vi "App - analyze RUS V6.vi"() -> ()   [LabVIEW 2021] (continued)
"mod time(min)"=58230516.86666667, "file format"=enum."binary", "power(V)"=2.1, "Magn Field(T) "=0.0}, {"temperature"=33.604, "temperature str"="33.60400", "file path"=path "D:/Data/Ultrasound/LSCO/LSCO22__130814c/5_Cooling_2nd_try/September_2014/091714/33.60400K_500_2500_2.10000V_0.00000T_Sep17-2014__16-38-11_001_091714.bin", "last mod"=timestamp(3493831091 s since 1904-01-01), "file name str"="D:\\Data\\Ultrasound\\LSCO\\LSCO22__130814c\\5_Cooling_2nd_try\\September_2014\\091714\\33.60400K_500_2500_2.10000V_0.00000T_Sep17-2014__16-38-11_001_091714.bin", "mod time(min)"=58230518.18333333, "file format"=enum."binary", "power(V)"=2.1, "Magn Field(T) "=0.0}, {"temperature"=33.517, "temperature str"="33.51700", "file path"=path "D:/Data/Ultrasound/LSCO/LSCO22__130814c/5_Cooling_2nd_try/September_2014/091714/33.51700K_500_2500_2.10000V_0.00000T_Sep17-2014__16-39-31_001_091714.bin", "last mod"=timestamp(3493831171 s since 1904-01-01), "file name str"="D:\\Data\\Ultrasound\\LSCO\\LSCO22__130814c\\5_Cooling_2nd_try\\September_2014\\091714\\33.51700K_500_2500_2.10000V_0.00000T_Sep17-2014__16-39-31_001_091714.bin", "mod time(min)"=58230519.516666666, "file format"=enum."binary", "power(V)"=2.1, "Magn Field(T) "=0.0}, {"temperature"=33.438, "temperature str"="33.43800", "file path"=path "D:/Data/Ultrasound/LSCO/LSCO22__130814c/5_Cooling_2nd_try/September_2014/091714/33.43800K_500_2500_2.10000V_0.00000T_Sep17-2014__16-40-50_001_091714.bin", "last mod"=timestamp(3493831250 s since 1904-01-01), "file name str"="D:\\Data\\Ultrasound\\LSCO\\LSCO22__130814c\\5_Cooling_2nd_try\\September_2014\\091714\\33.43800K_500_2500_2.10000V_0.00000T_Sep17-2014__16-40-50_001_091714.bin", "mod time(min)"=58230520.833333336, "file format"=enum."binary", "power(V)"=2.1, "Magn Field(T) "=0.0}, {"temperature"=33.342, "temperature str"="33.34200", "file path"=path "D:/Data/Ultrasound/LSCO/LSCO22__130814c/5_Cooling_2nd_try/September_2014/091714/33.34200K_500_2500_2.10000V_0.00000T_Sep17-2014__16-42-10_001_091714.bin", "last mod"=timestamp(3493831330 s since 1904-01-01), "file name str"="D:\\Data\\Ultrasound\\LSCO\\LSCO22__130814c\\5_Cooling_2nd_try\\September_2014\\091714\\33.34200K_500_2500_2.10000V_0.00000T_Sep17-2014__16-42-10_001_091714.bin", "mod time(min)"=58230522.166666664, "file format"=enum."binary", "power(V)"=2.1, "Magn Field(T) "=0.0}, {"temperature"=33.262, "temperature str"="33.26200", "file path"=path "D:/Data/Ultrasound/LSCO/LSCO22__130814c/5_Cooling_2nd_try/September_2014/091714/33.26200K_500_2500_2.10000V_0.00000T_Sep17-2014__16-43-29_001_091714.bin", "last mod"=timestamp(3493831409 s since 1904-01-01), "file name str"="D:\\Data\\Ultrasound\\LSCO\\LSCO22__130814c\\5_Cooling_2nd_try\\September_2014\\091714\\33.26200K_500_2500_2.10000V_0.00000T_Sep17-2014__16-43-29_001_091714.bin", "mod time(min)"=58230523.483333334, "file format"=enum."binary", "power(V)"=2.1, "Magn Field(T) "=0.0}, {"temperature"=33.17, "temperature str"="33.17000", "file path"=path "D:/Data/Ultrasound/LSCO/LSCO22__130814c/5_Cooling_2nd_try/September_2014/091714/33.17000K_500_2500_2.10000V_0.00000T_Sep17-2014__16-44-48_001_091714.bin", "last mod"=timestamp(3493831488 s since 1904-01-01), "file name str"="D:\\Data\\Ultrasound\\LSCO\\LSCO22__130814c\\5_Cooling_2nd_try\\September_2014\\091714\\33.17000K_500_2500_2.10000V_0.00000T_Sep17-2014__16-44-48_001_091714.bin", "mod time(min)"=58230524.8, "file format"=enum."binary", "power(V)"=2.1, "Magn Field(T) "=0.0}, {"temperature"=33.079, "temperature str"="33.07900", "file path"=path "D:/Data/Ultrasound/LSCO/LSCO22__130814c/5_Cooling_2nd_try/September_2014/091714/33.07900K_500_2500_2.10000V_0.00000T_Sep17-2014__16-46-08_001_091714.bin", "last mod"=timestamp(3493831568 s since 1904-01-01), "file name str"="D:\\Data\\Ultrasound\\LSCO\\LSCO22__130814c\\5_Cooling_2nd_try\\September_2014\\091714\\33.07900K_500_2500_2.10000V_0.00000T_Sep17-2014__16-46-08_001_091714.bin", "mod time(min)"=58230526.13333333, "file format"=enum."binary", "power(V)"=2.1, "Magn Field(T) "=0.0}, {"temperature"=32.992, "temperature str"="32.99200", "file path"=path "D:/Data/Ultrasound/LSCO/LSCO22__130814c/5_Cooling_2nd_try/September_2014/091714/32.99200K_500_2500_2.10000V_0.00000T_Sep17-2014__16-47-27_001_091714.bin", "last mod"=timestamp(3493831647 s since 1904-01-01), "file name str"="D:\\Data\\Ultrasound\\LSCO\\LSCO22__130814c\\5_Cooling_2nd_try\\September_2014\\091714\\32.99200K_500_2500_2.10000V_0.00000T_Sep17-2014__16-47-27_001_091714.bin", "mod time(min)"=58230527.45, "file format"=enum."binary", "power(V)"=2.1, "Magn Field(T) "=0.0}, {"temperature"=32.907, "temperature str"="32.90700", "file path"=path "D:/Data/Ultrasound/LSCO/LSCO22__130814c/5_Cooling_2nd_try/September_2014/091714/32.90700K_500_2500_2.10000V_0.00000T_Sep17-2014__16-48-46_001_091714.bin", "last mod"=timestamp(3493831726 s since 1904-01-01), "file name str"="D:\\Data\\Ultrasound\\LSCO\\LSCO22__130814c\\5_Cooling_2nd_try\\September_2014\\091714\\32.90700K_500_2500_2.10000V_0.00000T_Sep17-2014__16-48-46_001_091714.bin", "mod time(min)"=58230528.766666666, "file format"=enum."binary", "power(V)"=2.1, "Magn Field(T) "=0.0}, {"temperature"=32.817, "temperature str"="32.81700", "file path"=path "D:/Data/Ultrasound/LSCO/LSCO22__130814c/5_Cooling_2nd_try/September_2014/091714/32.81700K_500_2500_2.10000V_0.00000T_Sep17-2014__16-50-06_001_091714.bin", "last mod"=timestamp(3493831806 s since 1904-01-01), "file name str"="D:\\Data\\Ultrasound\\LSCO\\LSCO22__130814c\\5_Cooling_2nd_try\\September_2014\\091714\\32.81700K_500_2500_2.10000V_0.00000T_Sep17-2014__16-50-06_001_091714.bin", "mod time(min)"=58230530.1, "file format"=enum."binary", "power(V)"=2.1, "Magn Field(T) "=0.0}, {"temperature"=32.723, "temperature str"="32.72300", "file path"=path "D:/Data/Ultrasound/LSCO/LSCO22__130814c/5_Cooling_2nd_try/September_2014/091714/32.72300K_500_2500_2.10000V_0.00000T_Sep17-2014__16-51-25_001_091714.bin", "last mod"=timestamp(3493831885 s since 1904-01-01), "file name str"="D:\\Data\\Ultrasound\\LSCO\\LSCO22__130814c\\5_Cooling_2nd_try\\September_2014\\091714\\32.72300K_500_2500_2.10000V_0.00000T_Sep17-2014__16-51-25_001_091714.bin", "mod time(min)"=58230531.416666664, "file format"=enum."binary", "power(V)"=2.1, "Magn Field(T) "=0.0}, {"temperature"=32.637, "temperature str"="32.63700", "file path"=path "D:/Data/Ultrasound/LSCO/LSCO22__130814c/5_Cooling_2nd_try/September_2014/091714/32.63700K_500_2500_2.10000V_0.00000T_Sep17-2014__16-52-45_001_091714.bin", "last mod"=timestamp(3493831965 s since 1904-01-01), "file name str"="D:\\Data\\Ultrasound\\LSCO\\LSCO22__130814c\\5_Cooling_2nd_try\\September_2014\\091714\\32.63700K_500_2500_2.10000V_0.00000T_Sep17-2014__16-52-45_001_091714.bin", "mod time(min)"=58230532.75, "file format"=enum."binary", "power(V)"=2.1, "Magn Field(T) "=0.0}, {"temperature"=32.55, "temperature str"="32.55000", "file path"=path "D:/Data/Ultrasound/LSCO/LSCO22__130814c/5_Cooling_2nd_try/September_2014/091714/32.55000K_500_2500_2.10000V_0.00000T_Sep17-2014__16-54-04_001_091714.bin", "last mod"=timestamp(3493832044 s since 1904-01-01), "file name str"="D:\\Data\\Ultrasound\\LSCO\\LSCO22__130814c\\5_Cooling_2nd_try\\September_2014\\091714\\32.55000K_500_2500_2.10000V_0.00000T_Sep17-2014__16-54-04_001_091714.bin", "mod time(min)"=58230534.06666667, "file format"=enum."binary", "power(V)"=2.1, "Magn Field(T) "=0.0}, {"temperature"=32.462, "temperature str"="32.46200", "file path"=path "D:/Data/Ultrasound/LSCO/LSCO22__130814c/5_Cooling_2nd_try/September_2014/091714/32.46200K_500_2500_2.10000V_0.00000T_Sep17-2014__16-55-23_001_091714.bin", "last mod"=timestamp(3493832123 s since 1904-01-01), "file name str"="D:\\Data\\Ultrasound\\LSCO\\LSCO22__130814c\\5_Cooling_2nd_try\\September_2014\\091714\\32.46200K_500_2500_2.10000V_0.00000T_Sep17-2014__16-55-23_001_091714.bin", "mod time(min)"=58230535.38333333, "file format"=enum."binary", "power(V)"=2.1, "Magn Field(T) "=0.0}, {"temperature"=32.371, "temperature str"="32.37100", "file path"=path "D:/Data/Ultrasound/LSCO/LSCO22__130814c/5_Cooling_2nd_try/September_2014/091714/32.37100K_500_2500_2.10000V_0.00000T_Sep17-2014__16-56-43_001_091714.bin", "last mod"=timestamp(3493832203 s since 1904-01-01), "file name str"="D:\\Data\\Ultrasound\\LSCO\\LSCO22__130814c\\5_Cooling_2nd_try\\September_2014\\091714\\32.37100K_500_2500_2.10000V_0.00000T_Sep17-2014__16-56-43_001_091714.bin", "mod time(min)"=58230536.71666667, "file format"=enum."binary", "power(V)"=2.1, "Magn Field(T) "=0.0}, {"temperature"=32.282, "temperature str"="32.28200", "file path"=path "D:/Data/Ultrasound/LSCO/LSCO22__130814c/5_Cooling_2nd_try/September_2014/091714/32.28200K_500_2500_2.10000V_0.00000T_Sep17-2014__16-58-02_001_091714.bin", "last mod"=timestamp(3493832282 s since 1904-01-01), "file name str"="D:\\Data\\Ultrasound\\LSCO\\LSCO22__130814c\\5_Cooling_2nd_try\\September_2014\\091714\\32.28200K_500_2500_2.10000V_0.00000T_Sep17-2014__16-58-02_001_091714.bin", "mod time(min)"=58230538.03333333, "file format"=enum."binary", "power(V)"=2.1, "Magn Field(T) "=0.0}, {"temperature"=32.189, "temperature str"="32.18900", "file path"=path "D:/Data/Ultrasound/LSCO/LSCO22__130814c/5_Cooling_2nd_try/September_2014/091714/32.18900K_500_2500_2.10000V_0.00000T_Sep17-2014__16-59-22_001_091714.bin", "last mod"=timestamp(3493832362 s since 1904-01-01), "file name str"="D:\\Data\\Ultrasound\\LSCO\\LSCO22__130814c\\5_Cooling_2nd_try\\September_2014\\091714\\32.18900K_500_2500_2.10000V_0.00000T_Sep17-2014__16-59-22_001_091714.bin", "mod time(min)"=58230539.36666667, "file format"=enum."binary", "power(V)"=2.1, "Magn Field(T) "=0.0}, {"temperature"=32.102, "temperature str"="32.10200", "file path"=path "D:/Data/Ultrasound/LSCO/LSCO22__130814c/5_Cooling_2nd_try/September_2014/091714/32.10200K_500_2500_2.10000V_0.00000T_Sep17-2014__17-00-41_001_091714.bin", "last mod"=timestamp(3493832441 s since 1904-01-01), "file name str"="D:\\Data\\Ultrasound\\LSCO\\LSCO22__130814c\\5_Cooling_2nd_try\\September_2014\\091714\\32.10200K_500_2500_2.10000V_0.00000T_Sep17-2014__17-00-41_001_091714.bin", "mod time(min)"=58230540.68333333, "file format"=enum."binary", "power(V)"=2.1, "Magn Field(T) "=0.0}, {"temperature"=32.008, "temperature str"="32.00800", "file path"=path "D:/Data/Ultrasound/LSCO/LSCO22__130814c/5_Cooling_2nd_try/September_2014/091714/32.00800K_500_2500_2.10000V_0.00000T_Sep17-2014__17-02-00_001_091714.bin", "last mod"=timestamp(3493832520 s since 1904-01-01), "file name str"="D:\\Data\\Ultrasound\\LSCO\\LSCO22__130814c\\5_Cooling_2nd_try\\September_2014\\091714\\32.00800K_500_2500_2.10000V_0.00000T_Sep17-2014__17-02-00_001_091714.bin", "mod time(min)"=58230542.0, "file format"=enum."binary", "power(V)"=2.1, "Magn Field(T) "=0.0}, {"temperature"=31.925, "temperature str"="31.92500", "file path"=path "D:/Data/Ultrasound/LSCO/LSCO22__130814c/5_Cooling_2nd_try/September_2014/091714/31.92500K_500_2500_2.10000V_0.00000T_Sep17-2014__17-03-20_001_091714.bin", "last mod"=timestamp(3493832600 s since 1904-01-01), "file name str"="D:\\Data\\Ultrasound\\LSCO\\LSCO22__130814c\\5_Cooling_2nd_try\\September_2014\\091714\\31.92500K_500_2500_2.10000V_0.00000T_Sep17-2014__17-03-20_001_091714.bin", "mod time(min)"=58230543.333333336, "file format"=enum."binary", "power(V)"=2.1, "Magn Field(T) "=0.0}, {"temperature"=31.83, "temperature str"="31.83000", "file path"=path "D:/Data/Ultrasound/LSCO/LSCO22__130814c/5_Cooling_2nd_try/September_2014/091714/31.83000K_500_2500_2.10000V_0.00000T_Sep17-2014__17-04-39_001_091714.bin", "last mod"=timestamp(3493832679 s since 1904-01-01), "file name str"="D:\\Data\\Ultrasound\\LSCO\\LSCO22__130814c\\5_Cooling_2nd_try\\September_2014\\091714\\31.83000K_500_2500_2.10000V_0.00000T_Sep17-2014__17-04-39_001_091714.bin", "mod time(min)"=58230544.65, "file format"=enum."binary", "power(V)"=2.1, "Magn Field(T) "=0.0}, {"temperature"=31.738, "temperature str"="31.73800", "file path"=path "D:/Data/Ultrasound/LSCO/LSCO22__130814c/5_Cooling_2nd_try/September_2014/091714/31.73800K_500_2500_2.10000V_0.00000T_Sep17-2014__17-05-58_001_091714.bin", "last mod"=timestamp(3493832758 s since 1904-01-01), "file name str"="D:\\Data\\Ultrasound\\LSCO\\LSCO22__130814c\\5_Cooling_2nd_try\\September_2014\\091714\\31.73800K_500_2500_2.10000V_0.00000T_Sep17-2014__17-05-58_001_091714.bin", "mod time(min)"=58230545.96666667, "file format"=enum."binary", "power(V)"=2.1, "Magn Field(T) "=0.0}, {"temperature"=31.653, "temperature str"="31.65300", "file path"=path "D:/Data/Ultrasound/LSCO/LSCO22__130814c/5_Cooling_2nd_try/September_2014/091714/31.65300K_500_2500_2.10000V_0.00000T_Sep17-2014__17-07-18_001_091714.bin", "last mod"=timestamp(3493832838 s since 1904-01-01), "file name str"="D:\\Data\\Ultrasound\\LSCO\\LSCO22__130814c\\5_Cooling_2nd_try\\September_2014\\091714\\31.65300K_500_2500_2.10000V_0.00000T_Sep17-2014__17-07-18_001_091714.bin", "mod time(min)"=58230547.3, "file format"=enum."binary", "power(V)"=2.1, "Magn Field(T) "=0.0}, {"temperature"=31.556, "temperature str"="31.55600", "file path"=path "D:/Data/Ultrasound/LSCO/LSCO22__130814c/5_Cooling_2nd_try/September_2014/091714/31.55600K_500_2500_2.10000V_0.00000T_Sep17-2014__17-08-37_001_091714.bin", "last mod"=timestamp(3493832917 s since 1904-01-01), "file name str"="D:\\Data\\Ultrasound\\LSCO\\LSCO22__130814c\\5_Cooling_2nd_try\\September_2014\\091714\\31.55600K_500_2500_2.10000V_0.00000T_Sep17-2014__17-08-37_001_091714.bin", "mod time(min)"=58230548.61666667, "file format"=enum."binary", "power(V)"=2.1, "Magn Field(T) "=0.0}, {"temperature"=31.463, "temperature str"="31.46300", "file path"=path "D:/Data/Ultrasound/LSCO/LSCO22__130814c/5_Cooling_2nd_try/September_2014/091714/31.46300K_500_2500_2.10000V_0.00000T_Sep17-2014__17-09-57_001_091714.bin", "last mod"=timestamp(3493832997 s since 1904-01-01), "file name str"="D:\\Data\\Ultrasound\\LSCO\\LSCO22__130814c\\5_Cooling_2nd_try\\September_2014\\091714\\31.46300K_500_2500_2.10000V_0.00000T_Sep17-2014__17-09-57_001_091714.bin", "mod time(min)"=58230549.95, "file format"=enum."binary", "power(V)"=2.1, "Magn Field(T) "=0.0}, {"temperature"=31.383, "temperature str"="31.38300", "file path"=path "D:/Data/Ultrasound/LSCO/LSCO22__130814c/5_Cooling_2nd_try/September_2014/091714/31.38300K_500_2500_2.10000V_0.00000T_Sep17-2014__17-11-16_001_091714.bin", "last mod"=timestamp(3493833076 s since 1904-01-01), "file name str"="D:\\Data\\Ultrasound\\LSCO\\LSCO22__130814c\\5_Cooling_2nd_try\\September_2014\\091714\\31.38300K_500_2500_2.10000V_0.00000T_Sep17-2014__17-11-16_001_091714.bin", "mod time(min)"=58230551.266666666, "file format"=enum."binary", "power(V)"=2.1, "Magn Field(T) "=0.0}, {"temperature"=31.282, "temperature str"="31.28200", "file path"=path "D:/Data/Ultrasound/LSCO/LSCO22__130814c/5_Cooling_2nd_try/September_2014/091714/31.28200K_500_2500_2.10000V_0.00000T_Sep17-2014__17-12-35_001_091714.bin", "last mod"=timestamp(3493833155 s since 1904-01-01), "file name str"="D:\\Data\\Ultrasound\\LSCO\\LSCO22__130814c\\5_Cooling_2nd_try\\September_2014\\091714\\31.28200K_500_2500_2.10000V_0.00000T_Sep17-2014__17-12-35_001_091714.bin", "mod time(min)"=58230552.583333336, "file format"=enum."binary", "power(V)"=2.1, "Magn Field(T) "=0.0}, {"temperature"=31.196, "temperature str"="31.19600", "file path"=path "D:/Data/Ultrasound/LSCO/LSCO22__130814c/5_Cooling_2nd_try/September_2014/091714/31.19600K_500_2500_2.10000V_0.00000T_Sep17-2014__17-13-55_001_091714.bin", "last mod"=timestamp(3493833235 s since 1904-01-01), "file name str"="D:\\Data\\Ultrasound\\LSCO\\LSCO22__130814c\\5_Cooling_2nd_try\\September_2014\\091714\\31.19600K_500_2500_2.10000V_0.00000T_Sep17-2014__17-13-55_001_091714.bin", "mod time(min)"=58230553.916666664, "file format"=enum."binary", "power(V)"=2.1, "Magn Field(T) "=0.0}, {"temperature"=31.111, "temperature str"="31.11100", "file path"=path "D:/Data/Ultrasound/LSCO/LSCO22__130814c/5_Cooling_2nd_try/September_2014/091714/31.11100K_500_2500_2.10000V_0.00000T_Sep17-2014__17-15-14_001_091714.bin", "last mod"=timestamp(3493833314 s since 1904-01-01), "file name str"="D:\\Data\\Ultrasound\\LSCO\\LSCO22__130814c\\5_Cooling_2nd_try\\September_2014\\091714\\31.11100K_500_2500_2.10000V_0.00000T_Sep17-2014__17-15-14_001_091714.bin", "mod time(min)"=58230555.233333334, "file format"=enum."binary", "power(V)"=2.1, "Magn Field(T) "=0.0}, {"temperature"=31.006, "temperature str"="31.00600", "file path"=path "D:/Data/Ultrasound/LSCO/LSCO22__130814c/5_Cooling_2nd_try/September_2014/091714/31.00600K_500_2500_2.10000V_0.00000T_Sep17-2014__17-16-33_001_091714.bin", "last mod"=timestamp(3493833393 s since 1904-01-01), "file name str"="D:\\Data\\Ultrasound\\LSCO\\LSCO22__130814c\\5_Cooling_2nd_try\\September_2014\\091714\\31.00600K_500_2500_2.10000V_0.00000T_Sep17-2014__17-16-33_001_091714.bin", "mod time(min)"=58230556.55, "file format"=enum."binary", "power(V)"=2.1, "Magn Field(T) "=0.0}, {"temperature"=30.926, "temperature str"="30.92600", "file path"=path "D:/Data/Ultrasound/LSCO/LSCO22__130814c/5_Cooling_2nd_try/September_2014/091714/30.92600K_500_2500_2.10000V_0.00000T_Sep17-2014__17-17-53_001_091714.bin", "last mod"=timestamp(3493833473 s since 1904-01-01), "file name str"="D:\\Data\\Ultrasound\\LSCO\\LSCO22__130814c\\5_Cooling_2nd_try\\September_2014\\091714\\30.92600K_500_2500_2.10000V_0.00000T_Sep17-2014__17-17-53_001_091714.bin", "mod time(min)"=58230557.88333333, "file format"=enum."binary", "power(V)"=2.1, "Magn Field(T) "=0.0}, {"temperature"=30.834, "temperature str"="30.83400", "file path"=path "D:/Data/Ultrasound/LSCO/LSCO22__130814c/5_Cooling_2nd_try/September_2014/091714/30.83400K_500_2500_2.10000V_0.00000T_Sep17-2014__17-19-12_001_091714.bin", "last mod"=timestamp(3493833552 s since 1904-01-01), "file name str"="D:\\Data\\Ultrasound\\LSCO\\LSCO22__130814c\\5_Cooling_2nd_try\\September_2014\\091714\\30.83400K_500_2500_2.10000V_0.00000T_Sep17-2014__17-19-12_001_091714.bin", "mod time(min)"=58230559.2, "file format"=enum."binary", "power(V)"=2.1, "Magn Field(T) "=0.0}, {"temperature"=30.738, "temperature str"="30.73800", "file path"=path "D:/Data/Ultrasound/LSCO/LSCO22__130814c/5_Cooling_2nd_try/September_2014/091714/30.73800K_500_2500_2.10000V_0.00000T_Sep17-2014__17-20-32_001_091714.bin", "last mod"=timestamp(3493833632 s since 1904-01-01), "file name str"="D:\\Data\\Ultrasound\\LSCO\\LSCO22__130814c\\5_Cooling_2nd_try\\September_2014\\091714\\30.73800K_500_2500_2.10000V_0.00000T_Sep17-2014__17-20-32_001_091714.bin", "mod time(min)"=58230560.53333333, "file format"=enum."binary", "power(V)"=2.1, "Magn Field(T) "=0.0}, {"temperature"=30.648, "temperature str"="30.64800", "file path"=path "D:/Data/Ultrasound/LSCO/LSCO22__130814c/5_Cooling_2nd_try/September_2014/091714/30.64800K_500_2500_2.10000V_0.00000T_Sep17-2014__17-21-51_001_091714.bin", "last mod"=timestamp(3493833711 s since 1904-01-01), "file name str"="D:\\Data\\Ultrasound\\LSCO\\LSCO22__130814c\\5_Cooling_2nd_try\\September_2014\\091714\\30.64800K_500_2500_2.10000V_0.00000T_Sep17-2014__17-21-51_001_091714.bin", "mod time(min)"=58230561.85, "file format"=enum."binary", "power(V)"=2.1, "Magn Field(T) "=0.0}, {"temperature"=30.563, "temperature str"="30.56300", "file path"=path "D:/Data/Ultrasound/LSCO/LSCO22__130814c/5_Cooling_2nd_try/September_2014/091714/30.56300K_500_2500_2.10000V_0.00000T_Sep17-2014__17-23-10_001_091714.bin", "last mod"=timestamp(3493833790 s since 1904-01-01), "file name str"="D:\\Data\\Ultrasound\\LSCO\\LSCO22__130814c\\5_Cooling_2nd_try\\September_2014\\091714\\30.56300K_500_2500_2.10000V_0.00000T_Sep17-2014__17-23-10_001_091714.bin", "mod time(min)"=58230563.166666664, "file format"=enum."binary", "power(V)"=2.1, "Magn Field(T) "=0.0}, {"temperature"=30.467, "temperature str"="30.46700", "file path"=path "D:/Data/Ultrasound/LSCO/LSCO22__130814c/5_Cooling_2nd_try/September_2014/091714/30.46700K_500_2500_2.10000V_0.00000T_Sep17-2014__17-24-30_001_091714.bin", "last mod"=timestamp(3493833870 s since 1904-01-01), "file name str"="D:\\Data\\Ultrasound\\LSCO\\LSCO22__130814c\\5_Cooling_2nd_try\\September_2014\\091714\\30.46700K_500_2500_2.10000V_0.00000T_Sep17-2014__17-24-30_001_091714.bin", "mod time(min)"=58230564.5, "file format"=enum."binary", "power(V)"=2.1, "Magn Field(T) "=0.0}, {"temperature"=30.376, "temperature str"="30.37600", "file path"=path "D:/Data/Ultrasound/LSCO/LSCO22__130814c/5_Cooling_2nd_try/September_2014/091714/30.37600K_500_2500_2.10000V_0.00000T_Sep17-2014__17-25-49_001_091714.bin", "last mod"=timestamp(3493833949 s since 1904-01-01), "file name str"="D:\\Data\\Ultrasound\\LSCO\\LSCO22__130814c\\5_Cooling_2nd_try\\September_2014\\091714\\30.37600K_500_2500_2.10000V_0.00000T_Sep17-2014__17-25-49_001_091714.bin", "mod time(min)"=58230565.81666667, "file format"=enum."binary", "power(V)"=2.1, "Magn Field(T) "=0.0}, {"temperature"=30.285, "temperature str"="30.28500", "file path"=path "D:/Data/Ultrasound/LSCO/LSCO22__130814c/5_Cooling_2nd_try/September_2014/091714/30.28500K_500_2500_2.10000V_0.00000T_Sep17-2014__17-27-09_001_091714.bin", "last mod"=timestamp(3493834029 s since 1904-01-01), "file name str"="D:\\Data\\Ultrasound\\LSCO\\LSCO22__130814c\\5_Cooling_2nd_try\\September_2014\\091714\\30.28500K_500_2500_2.10000V_0.00000T_Sep17-2014__17-27-09_001_091714.bin", "mod time(min)"=58230567.15, "file format"=enum."binary", "power(V)"=2.1, "Magn Field(T) "=0.0}, {"temperature"=30.196, "temperature str"="30.19600", "file path"=path "D:/Data/Ultrasound/LSCO/LSCO22__130814c/5_Cooling_2nd_try/September_2014/091714/30.19600K_500_2500_2.10000V_0.00000T_Sep17-2014__17-28-28_001_091714.bin", "last mod"=timestamp(3493834108 s since 1904-01-01), "file name str"="D:\\Data\\Ultrasound\\LSCO\\LSCO22__130814c\\5_Cooling_2nd_try\\September_2014\\091714\\30.19600K_500_2500_2.10000V_0.00000T_Sep17-2014__17-28-28_001_091714.bin", "mod time(min)"=58230568.46666667, "file format"=enum."binary", "power(V)"=2.1, "Magn Field(T) "=0.0}, {"temperature"=30.104, "temperature str"="30.10400", "file path"=path "D:/Data/Ultrasound/LSCO/LSCO22__130814c/5_Cooling_2nd_try/September_2014/091714/30.10400K_500_2500_2.10000V_0.00000T_Sep17-2014__17-29-47_001_091714.bin", "last mod"=timestamp(3493834187 s since 1904-01-01), "file name str"="D:\\Data\\Ultrasound\\LSCO\\LSCO22__130814c\\5_Cooling_2nd_try\\September_2014\\091714\\30.10400K_500_2500_2.10000V_0.00000T_Sep17-2014__17-29-47_001_091714.bin", "mod time(min)"=58230569.78333333, "file format"=enum."binary", "power(V)"=2.1, "Magn Field(T) "=0.0}, {"temperature"=30.009, "temperature str"="30.00900", "file path"=path "D:/Data/Ultrasound/LSCO/LSCO22__130814c/5_Cooling_2nd_try/September_2014/091714/30.00900K_500_2500_2.10000V_0.00000T_Sep17-2014__17-31-07_001_091714.bin", "last mod"=timestamp(3493834267 s since 1904-01-01), "file name str"="D:\\Data\\Ultrasound\\LSCO\\LSCO22__130814c\\5_Cooling_2nd_try\\September_2014\\091714\\30.00900K_500_2500_2.10000V_0.00000T_Sep17-2014__17-31-07_001_091714.bin", "mod time(min)"=58230571.11666667, "file format"=enum."binary", "power(V)"=2.1, "Magn Field(T) "=0.0}, {"temperature"=29.914, "temperature str"="29.91400", "file path"=path "D:/Data/Ultrasound/LSCO/LSCO22__130814c/5_Cooling_2nd_try/September_2014/091714/29.91400K_500_2500_2.10000V_0.00000T_Sep17-2014__17-32-26_001_091714.bin", "last mod"=timestamp(3493834346 s since 1904-01-01), "file name str"="D:\\Data\\Ultrasound\\LSCO\\LSCO22__130814c\\5_Cooling_2nd_try\\September_2014\\091714\\29.91400K_500_2500_2.10000V_0.00000T_Sep17-2014__17-32-26_001_091714.bin", "mod time(min)"=58230572.43333333, "file format"=enum."binary", "power(V)"=2.1, "Magn Field(T) "=0.0}, {"temperature"=29.832, "temperature str"="29.83200", "file path"=path "D:/Data/Ultrasound/LSCO/LSCO22__130814c/5_Cooling_2nd_try/September_2014/091714/29.83200K_500_2500_2.10000V_0.00000T_Sep17-2014__17-33-45_001_091714.bin", "last mod"=timestamp(3493834425 s since 1904-01-01), "file name str"="D:\\Data\\Ultrasound\\LSCO\\LSCO22__130814c\\5_Cooling_2nd_try\\September_2014\\091714\\29.83200K_500_2500_2.10000V_0.00000T_Sep17-2014__17-33-45_001_091714.bin", "mod time(min)"=58230573.75, "file format"=enum."binary", "power(V)"=2.1, "Magn Field(T) "=0.0}, {"temperature"=29.737, "temperature str"="29.73700", "file path"=path "D:/Data/Ultrasound/LSCO/LSCO22__130814c/5_Cooling_2nd_try/September_2014/091714/29.73700K_500_2500_2.10000V_0.00000T_Sep17-2014__17-35-05_001_091714.bin", "last mod"=timestamp(3493834505 s since 1904-01-01), "file name str"="D:\\Data\\Ultrasound\\LSCO\\LSCO22__130814c\\5_Cooling_2nd_try\\September_2014\\091714\\29.73700K_500_2500_2.10000V_0.00000T_Sep17-2014__17-35-05_001_091714.bin", "mod time(min)"=58230575.083333336, "file format"=enum."binary", "power(V)"=2.1, "Magn Field(T) "=0.0}, {"temperature"=29.637, "temperature str"="29.63700", "file path"=path "D:/Data/Ultrasound/LSCO/LSCO22__130814c/5_Cooling_2nd_try/September_2014/091714/29.63700K_500_2500_2.10000V_0.00000T_Sep17-2014__17-36-24_001_091714.bin", "last mod"=timestamp(3493834584 s since 1904-01-01), "file name str"="D:\\Data\\Ultrasound\\LSCO\\LSCO22__130814c\\5_Cooling_2nd_try\\September_2014\\091714\\29.63700K_500_2500_2.10000V_0.00000T_Sep17-2014__17-36-24_001_091714.bin", "mod time(min)"=58230576.4, "file format"=enum."binary", "power(V)"=2.1, "Magn Field(T) "=0.0}, {"temperature"=29.553, "temperature str"="29.55300", "file path"=path "D:/Data/Ultrasound/LSCO/LSCO22__130814c/5_Cooling_2nd_try/September_2014/091714/29.55300K_500_2500_2.10000V_0.00000T_Sep17-2014__17-37-44_001_091714.bin", "last mod"=timestamp(3493834664 s since 1904-01-01), "file name str"="D:\\Data\\Ultrasound\\LSCO\\LSCO22__130814c\\5_Cooling_2nd_try\\September_2014\\091714\\29.55300K_500_2500_2.10000V_0.00000T_Sep17-2014__17-37-44_001_091714.bin", "mod time(min)"=58230577.733333334, "file format"=enum."binary", "power(V)"=2.1, "Magn Field(T) "=0.0}, {"temperature"=29.453, "temperature str"="29.45300", "file path"=path "D:/Data/Ultrasound/LSCO/LSCO22__130814c/5_Cooling_2nd_try/September_2014/091714/29.45300K_500_2500_2.10000V_0.00000T_Sep17-2014__17-39-03_001_091714.bin", "last mod"=timestamp(3493834743 s since 1904-01-01), "file name str"="D:\\Data\\Ultrasound\\LSCO\\LSCO22__130814c\\5_Cooling_2nd_try\\September_2014\\091714\\29.45300K_500_2500_2.10000V_0.00000T_Sep17-2014__17-39-03_001_091714.bin", "mod time(min)"=58230579.05, "file format"=enum."binary", "power(V)"=2.1, "Magn Field(T) "=0.0}, {"temperature"=29.362, "temperature str"="29.36200", "file path"=path "D:/Data/Ultrasound/LSCO/LSCO22__130814c/5_Cooling_2nd_try/September_2014/091714/29.36200K_500_2500_2.10000V_0.00000T_Sep17-2014__17-40-22_001_091714.bin", "last mod"=timestamp(3493834822 s since 1904-01-01), "file name str"="D:\\Data\\Ultrasound\\LSCO\\LSCO22__130814c\\5_Cooling_2nd_try\\September_2014\\091714\\29.36200K_500_2500_2.10000V_0.00000T_Sep17-2014__17-40-22_001_091714.bin", "mod time(min)"=58230580.36666667, "file format"=enum."binary", "power(V)"=2.1, "Magn Field(T) "=0.0}, {"temperature"=29.272, "temperature str"="29.27200", "file path"=path "D:/Data/Ultrasound/LSCO/LSCO22__130814c/5_Cooling_2nd_try/September_2014/091714/29.27200K_500_2500_2.10000V_0.00000T_Sep17-2014__17-41-42_001_091714.bin", "last mod"=timestamp(3493834902 s since 1904-01-01), "file name str"="D:\\Data\\Ultrasound\\LSCO\\LSCO22__130814c\\5_Cooling_2nd_try\\September_2014\\091714\\29.27200K_500_2500_2.10000V_0.00000T_Sep17-2014__17-41-42_001_091714.bin", "mod time(min)"=58230581.7, "file format"=enum."binary", "power(V)"=2.1, "Magn Field(T) "=0.0}, {"temperature"=29.18, "temperature str"="29.18000", "file path"=path "D:/Data/Ultrasound/LSCO/LSCO22__130814c/5_Cooling_2nd_try/September_2014/091714/29.18000K_500_2500_2.10000V_0.00000T_Sep17-2014__17-43-01_001_091714.bin", "last mod"=timestamp(3493834981 s since 1904-01-01), "file name str"="D:\\Data\\Ultrasound\\LSCO\\LSCO22__130814c\\5_Cooling_2nd_try\\September_2014\\091714\\29.18000K_500_2500_2.10000V_0.00000T_Sep17-2014__17-43-01_001_091714.bin", "mod time(min)"=58230583.016666666, "file format"=enum."binary", "power(V)"=2.1, "Magn Field(T) "=0.0}, {"temperature"=29.085, "temperature str"="29.08500", "file path"=path "D:/Data/Ultrasound/LSCO/LSCO22__130814c/5_Cooling_2nd_try/September_2014/091714/29.08500K_500_2500_2.10000V_0.00000T_Sep17-2014__17-44-21_001_091714.bin", "last mod"=timestamp(3493835061 s since 1904-01-01), "file name str"="D:\\Data\\Ultrasound\\LSCO\\LSCO22__130814c\\5_Cooling_2nd_try\\September_2014\\091714\\29.08500K_500_2500_2.10000V_0.00000T_Sep17-2014__17-44-21_001_091714.bin", "mod time(min)"=58230584.35, "file format"=enum."binary", "power(V)"=2.1, "Magn Field(T) "=0.0}, {"temperature"=28.992, "temperature str"="28.99200", "file path"=path "D:/Data/Ultrasound/LSCO/LSCO22__130814c/5_Cooling_2nd_try/September_2014/091714/28.99200K_500_2500_2.10000V_0.00000T_Sep17-2014__17-45-40_001_091714.bin", "last mod"=timestamp(3493835140 s since 1904-01-01), "file name str"="D:\\Data\\Ultrasound\\LSCO\\LSCO22__130814c\\5_Cooling_2nd_try\\September_2014\\091714\\28.99200K_500_2500_2.10000V_0.00000T_Sep17-2014__17-45-40_001_091714.bin", "mod time(min)"=58230585.666666664, "file format"=enum."binary", "power(V)"=2.1, "Magn Field(T) "=0.0}, {"temperature"=28.892, "temperature str"="28.89200", "file path"=path "D:/Data/Ultrasound/LSCO/LSCO22__130814c/5_Cooling_2nd_try/September_2014/091714/28.89200K_500_2500_2.10000V_0.00000T_Sep17-2014__17-46-59_001_091714.bin", "last mod"=timestamp(3493835219 s since 1904-01-01), "file name str"="D:\\Data\\Ultrasound\\LSCO\\LSCO22__130814c\\5_Cooling_2nd_try\\September_2014\\091714\\28.89200K_500_2500_2.10000V_0.00000T_Sep17-2014__17-46-59_001_091714.bin", "mod time(min)"=58230586.983333334, "file format"=enum."binary", "power(V)"=2.1, "Magn Field(T) "=0.0}, {"temperature"=28.803, "temperature str"="28.80300", "file path"=path "D:/Data/Ultrasound/LSCO/LSCO22__130814c/5_Cooling_2nd_try/September_2014/091714/28.80300K_500_2500_2.10000V_0.00000T_Sep17-2014__17-48-19_001_091714.bin", "last mod"=timestamp(3493835299 s since 1904-01-01), "file name str"="D:\\Data\\Ultrasound\\LSCO\\LSCO22__130814c\\5_Cooling_2nd_try\\September_2014\\091714\\28.80300K_500_2500_2.10000V_0.00000T_Sep17-2014__17-48-19_001_091714.bin", "mod time(min)"=58230588.31666667, "file format"=enum."binary", "power(V)"=2.1, "Magn Field(T) "=0.0}, {"temperature"=28.71, "temperature str"="28.71000", "file path"=path "D:/Data/Ultrasound/LSCO/LSCO22__130814c/5_Cooling_2nd_try/September_2014/091714/28.71000K_500_2500_2.10000V_0.00000T_Sep17-2014__17-49-38_001_091714.bin", "last mod"=timestamp(3493835378 s since 1904-01-01), "file name str"="D:\\Data\\Ultrasound\\LSCO\\LSCO22__130814c\\5_Cooling_2nd_try\\September_2014\\091714\\28.71000K_500_2500_2.10000V_0.00000T_Sep17-2014__17-49-38_001_091714.bin", "mod time(min)"=58230589.63333333, "file format"=enum."binary", "power(V)"=2.1, "Magn Field(T) "=0.0}, {"temperature"=28.614, "temperature str"="28.61400", "file path"=path "D:/Data/Ultrasound/LSCO/LSCO22__130814c/5_Cooling_2nd_try/September_2014/091714/28.61400K_500_2500_2.10000V_0.00000T_Sep17-2014__17-50-57_001_091714.bin", "last mod"=timestamp(3493835457 s since 1904-01-01), "file name str"="D:\\Data\\Ultrasound\\LSCO\\LSCO22__130814c\\5_Cooling_2nd_try\\September_2014\\091714\\28.61400K_500_2500_2.10000V_0.00000T_Sep17-2014__17-50-57_001_091714.bin", "mod time(min)"=58230590.95, "file format"=enum."binary", "power(V)"=2.1, "Magn Field(T) "=0.0}, {"temperature"=28.52, "temperature str"="28.52000", "file path"=path "D:/Data/Ultrasound/LSCO/LSCO22__130814c/5_Cooling_2nd_try/September_2014/091714/28.52000K_500_2500_2.10000V_0.00000T_Sep17-2014__17-52-17_001_091714.bin", "last mod"=timestamp(3493835537 s since 1904-01-01), "file name str"="D:\\Data\\Ultrasound\\LSCO\\LSCO22__130814c\\5_Cooling_2nd_try\\September_2014\\091714\\28.52000K_500_2500_2.10000V_0.00000T_Sep17-2014__17-52-17_001_091714.bin", "mod time(min)"=58230592.28333333, "file format"=enum."binary", "power(V)"=2.1, "Magn Field(T) "=0.0}, {"temperature"=28.426, "temperature str"="28.42600", "file path"=path "D:/Data/Ultrasound/LSCO/LSCO22__130814c/5_Cooling_2nd_try/September_2014/091714/28.42600K_500_2500_2.10000V_0.00000T_Sep17-2014__17-53-36_001_091714.bin", "last mod"=timestamp(3493835616 s since 1904-01-01), "file name str"="D:\\Data\\Ultrasound\\LSCO\\LSCO22__130814c\\5_Cooling_2nd_try\\September_2014\\091714\\28.42600K_500_2500_2.10000V_0.00000T_Sep17-2014__17-53-36_001_091714.bin", "mod time(min)"=58230593.6, "file format"=enum."binary", "power(V)"=2.1, "Magn Field(T) "=0.0}, {"temperature"=28.336, "temperature str"="28.33600", "file path"=path "D:/Data/Ultrasound/LSCO/LSCO22__130814c/5_Cooling_2nd_try/September_2014/091714/28.33600K_500_2500_2.10000V_0.00000T_Sep17-2014__17-54-56_001_091714.bin", "last mod"=timestamp(3493835696 s since 1904-01-01), "file name str"="D:\\Data\\Ultrasound\\LSCO\\LSCO22__130814c\\5_Cooling_2nd_try\\September_2014\\091714\\28.33600K_500_2500_2.10000V_0.00000T_Sep17-2014__17-54-56_001_091714.bin", "mod time(min)"=58230594.93333333, "file format"=enum."binary", "power(V)"=2.1, "Magn Field(T) "=0.0}, {"temperature"=28.239, "temperature str"="28.23900", "file path"=path "D:/Data/Ultrasound/LSCO/LSCO22__130814c/5_Cooling_2nd_try/September_2014/091714/28.23900K_500_2500_2.10000V_0.00000T_Sep17-2014__17-56-15_001_091714.bin", "last mod"=timestamp(3493835775 s since 1904-01-01), "file name str"="D:\\Data\\Ultrasound\\LSCO\\LSCO22__130814c\\5_Cooling_2nd_try\\September_2014\\091714\\28.23900K_500_2500_2.10000V_0.00000T_Sep17-2014__17-56-15_001_091714.bin", "mod time(min)"=58230596.25, "file format"=enum."binary", "power(V)"=2.1, "Magn Field(T) "=0.0}, {"temperature"=28.151, "temperature str"="28.15100", "file path"=path "D:/Data/Ultrasound/LSCO/LSCO22__130814c/5_Cooling_2nd_try/September_2014/091714/28.15100K_500_2500_2.10000V_0.00000T_Sep17-2014__17-57-34_001_091714.bin", "last mod"=timestamp(3493835854 s since 1904-01-01), "file name str"="D:\\Data\\Ultrasound\\LSCO\\LSCO22__130814c\\5_Cooling_2nd_try\\September_2014\\091714\\28.15100K_500_2500_2.10000V_0.00000T_Sep17-2014__17-57-34_001_091714.bin", "mod time(min)"=58230597.56666667, "file format"=enum."binary", "power(V)"=2.1, "Magn Field(T) "=0.0}, {"temperature"=28.051, "temperature str"="28.05100", "file path"=path "D:/Data/Ultrasound/LSCO/LSCO22__130814c/5_Cooling_2nd_try/September_2014/091714/28.05100K_500_2500_2.10000V_0.00000T_Sep17-2014__17-58-54_001_091714.bin", "last mod"=timestamp(3493835934 s since 1904-01-01), "file name str"="D:\\Data\\Ultrasound\\LSCO\\LSCO22__130814c\\5_Cooling_2nd_try\\September_2014\\091714\\28.05100K_500_2500_2.10000V_0.00000T_Sep17-2014__17-58-54_001_091714.bin", "mod time(min)"=58230598.9, "file format"=enum."binary", "power(V)"=2.1, "Magn Field(T) "=0.0}, {"temperature"=27.959, "temperature str"="27.95900", "file path"=path "D:/Data/Ultrasound/LSCO/LSCO22__130814c/5_Cooling_2nd_try/September_2014/091714/27.95900K_500_2500_2.10000V_0.00000T_Sep17-2014__18-00-13_001_091714.bin", "last mod"=timestamp(3493836013 s since 1904-01-01), "file name str"="D:\\Data\\Ultrasound\\LSCO\\LSCO22__130814c\\5_Cooling_2nd_try\\September_2014\\091714\\27.95900K_500_2500_2.10000V_0.00000T_Sep17-2014__18-00-13_001_091714.bin", "mod time(min)"=58230600.21666667, "file format"=enum."binary", "power(V)"=2.1, "Magn Field(T) "=0.0}, {"temperature"=27.87, "temperature str"="27.87000", "file path"=path "D:/Data/Ultrasound/LSCO/LSCO22__130814c/5_Cooling_2nd_try/September_2014/091714/27.87000K_500_2500_2.10000V_0.00000T_Sep17-2014__18-01-32_001_091714.bin", "last mod"=timestamp(3493836092 s since 1904-01-01), "file name str"="D:\\Data\\Ultrasound\\LSCO\\LSCO22__130814c\\5_Cooling_2nd_try\\September_2014\\091714\\27.87000K_500_2500_2.10000V_0.00000T_Sep17-2014__18-01-32_001_091714.bin", "mod time(min)"=58230601.53333333, "file format"=enum."binary", "power(V)"=2.1, "Magn Field(T) "=0.0}, {"temperature"=27.768, "temperature str"="27.76800", "file path"=path "D:/Data/Ultrasound/LSCO/LSCO22__130814c/5_Cooling_2nd_try/September_2014/091714/27.76800K_500_2500_2.10000V_0.00000T_Sep17-2014__18-02-52_001_091714.bin", "last mod"=timestamp(3493836172 s since 1904-01-01), "file name str"="D:\\Data\\Ultrasound\\LSCO\\LSCO22__130814c\\5_Cooling_2nd_try\\September_2014\\091714\\27.76800K_500_2500_2.10000V_0.00000T_Sep17-2014__18-02-52_001_091714.bin", "mod time(min)"=58230602.86666667, "file format"=enum."binary", "power(V)"=2.1, "Magn Field(T) "=0.0}, {"temperature"=27.675, "temperature str"="27.67500", "file path"=path "D:/Data/Ultrasound/LSCO/LSCO22__130814c/5_Cooling_2nd_try/September_2014/091714/27.67500K_500_2500_2.10000V_0.00000T_Sep17-2014__18-04-11_001_091714.bin", "last mod"=timestamp(3493836251 s since 1904-01-01), "file name str"="D:\\Data\\Ultrasound\\LSCO\\LSCO22__130814c\\5_Cooling_2nd_try\\September_2014\\091714\\27.67500K_500_2500_2.10000V_0.00000T_Sep17-2014__18-04-11_001_091714.bin", "mod time(min)"=58230604.18333333, "file format"=enum."binary", "power(V)"=2.1, "Magn Field(T) "=0.0}, {"temperature"=27.583, "temperature str"="27.58300", "file path"=path "D:/Data/Ultrasound/LSCO/LSCO22__130814c/5_Cooling_2nd_try/September_2014/091714/27.58300K_500_2500_2.10000V_0.00000T_Sep17-2014__18-05-31_001_091714.bin", "last mod"=timestamp(3493836331 s since 1904-01-01), "file name str"="D:\\Data\\Ultrasound\\LSCO\\LSCO22__130814c\\5_Cooling_2nd_try\\September_2014\\091714\\27.58300K_500_2500_2.10000V_0.00000T_Sep17-2014__18-05-31_001_091714.bin", "mod time(min)"=58230605.516666666, "file format"=enum."binary", "power(V)"=2.1, "Magn Field(T) "=0.0}, {"temperature"=27.483, "temperature str"="27.48300", "file path"=path "D:/Data/Ultrasound/LSCO/LSCO22__130814c/5_Cooling_2nd_try/September_2014/091714/27.48300K_500_2500_2.10000V_0.00000T_Sep17-2014__18-06-50_001_091714.bin", "last mod"=timestamp(3493836410 s since 1904-01-01), "file name str"="D:\\Data\\Ultrasound\\LSCO\\LSCO22__130814c\\5_Cooling_2nd_try\\September_2014\\091714\\27.48300K_500_2500_2.10000V_0.00000T_Sep17-2014__18-06-50_001_091714.bin", "mod time(min)"=58230606.833333336, "file format"=enum."binary", "power(V)"=2.1, "Magn Field(T) "=0.0}, {"temperature"=27.396, "temperature str"="27.39600", "file path"=path "D:/Data/Ultrasound/LSCO/LSCO22__130814c/5_Cooling_2nd_try/September_2014/091714/27.39600K_500_2500_2.10000V_0.00000T_Sep17-2014__18-08-09_001_091714.bin", "last mod"=timestamp(3493836489 s since 1904-01-01), "file name str"="D:\\Data\\Ultrasound\\LSCO\\LSCO22__130814c\\5_Cooling_2nd_try\\September_2014\\091714\\27.39600K_500_2500_2.10000V_0.00000T_Sep17-2014__18-08-09_001_091714.bin", "mod time(min)"=58230608.15, "file format"=enum."binary", "power(V)"=2.1, "Magn Field(T) "=0.0}, {"temperature"=27.297, "temperature str"="27.29700", "file path"=path "D:/Data/Ultrasound/LSCO/LSCO22__130814c/5_Cooling_2nd_try/September_2014/091714/27.29700K_500_2500_2.10000V_0.00000T_Sep17-2014__18-09-29_001_091714.bin", "last mod"=timestamp(3493836569 s since 1904-01-01), "file name str"="D:\\Data\\Ultrasound\\LSCO\\LSCO22__130814c\\5_Cooling_2nd_try\\September_2014\\091714\\27.29700K_500_2500_2.10000V_0.00000T_Sep17-2014__18-09-29_001_091714.bin", "mod time(min)"=58230609.483333334, "file format"=enum."binary", "power(V)"=2.1, "Magn Field(T) "=0.0}, {"temperature"=27.202, "temperature str"="27.20200", "file path"=path "D:/Data/Ultrasound/LSCO/LSCO22__130814c/5_Cooling_2nd_try/September_2014/091714/27.20200K_500_2500_2.10000V_0.00000T_Sep17-2014__18-10-48_001_091714.bin", "last mod"=timestamp(3493836648 s since 1904-01-01), "file name str"="D:\\Data\\Ultrasound\\LSCO\\LSCO22__130814c\\5_Cooling_2nd_try\\September_2014\\091714\\27.20200K_500_2500_2.10000V_0.00000T_Sep17-2014__18-10-48_001_091714.bin", "mod time(min)"=58230610.8, "file format"=enum."binary", "power(V)"=2.1, "Magn Field(T) "=0.0}, {"temperature"=27.113, "temperature str"="27.11300", "file path"=path "D:/Data/Ultrasound/LSCO/LSCO22__130814c/5_Cooling_2nd_try/September_2014/091714/27.11300K_500_2500_2.10000V_0.00000T_Sep17-2014__18-12-08_001_091714.bin", 
